vi "I2C Read.vi"(0 "handle":u32, 1 "options":u32, 5 "buffer":string, 7 "sizeToTransfer":u32, 9 "sizeTransfered":u32, 11 "error in (no error)":errorcluster) -> (4 "handle out":u32, 6 "buffer out":string, 8 "function return":u32, 10 "sizeTransfered out":u32, 15 "error out":errorcluster)   [LabVIEW 2024, in "libMPSSE-I2C.lvlib"]
doc: "FTDI_API FT_STATUS SPI_Read(FT_HANDLE handle, uint8 *buffer,\n uint32 sizeToTransfer, uint32 *sizeTransfered, uint32 options);"
uses:
  libMPSSE-I2C.lvlib
  libmpsse.dll
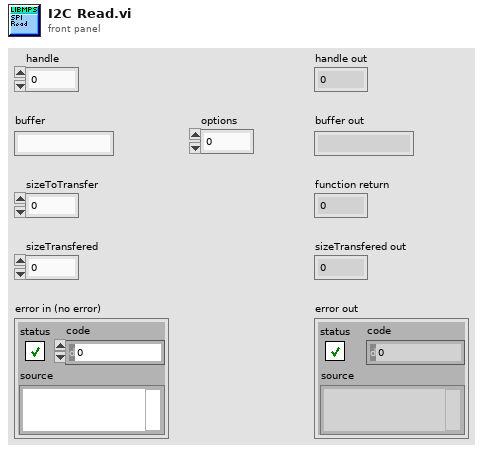
[diagram p1: front panel]
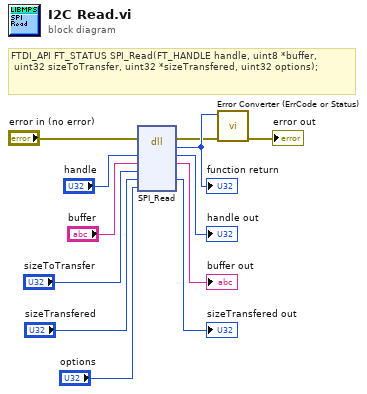
[diagram p0: block diagram]
diagram:
  # "FTDI_API FT_STATUS SPI_Read(FT_HANDLE handle, uint8 *buffer,\n\tuint32 sizeToTransfer, uint32 *sizeTransfered, uint32 options);"
  n1 = dll-call lib="C:/Workspace/sm_6576_001_RIB_Sequencer/I2C/libMPSSE.*" fn="SPI_Read"(error in="error in (no error)", "handle"="handle", "buffer"="buffer", "sizeToTransfer"="sizeToTransfer", "sizeTransfered"="sizeTransfered", "options"="options") -> (error out=w2:errorcluster, w12:u32, "handle"=→"handle out":u32, "buffer"=→"buffer out":string, "sizeTransfered"=→"sizeTransfered out":u32)  [unwired: 4 in, 1 out]
  "function return" <- w12
  n2 = call "Error Converter (ErrCode or Status).vi"("error in (no error)"=w2, "error code"=w12) -> ("error out"=→"error out":errorcluster)  [unwired: 9 in]
